vi "Decrypt_Selected_File_of_Hierarchy_Data.vi"(8 "error in (no error)":errorcluster, 9 "FileName":string, 10 "SubFolderName":string, 11 "object in":refnum<class "Crypter.lvclass">) -> (0 "error out":errorcluster, 1 "Folder_Mgmt out":refnum<class "Folder_Mgmt.lvclass">, 2 "Dencrypted text":string, 3 "object out":refnum<class "Crypter.lvclass">)   [LabVIEW 2016, in "Crypter.lvclass"]
uses:
  Crypter.lvclass
  C:/Users/Marco Preziani/Documents/DOME-LV16/WebBrowser_Mgmt/WebBrowser_Mgmt.lvclass
  Folder_Mgmt/Folder_Mgmt.lvclass
  WebBrowser_Mgmt/WebBrowser_Mgmt.lvclass/WebBrowser_Mgmt.ctl
  Folder_Mgmt/Folder_Mgmt.lvclass/Folder_Mgmt.ctl
  WebBrowser_Mgmt/WebBrowser_Mgmt.lvclass
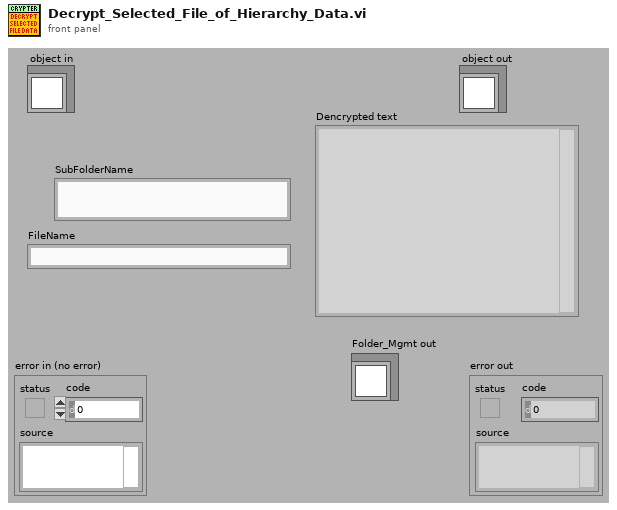
[diagram p1: front panel]
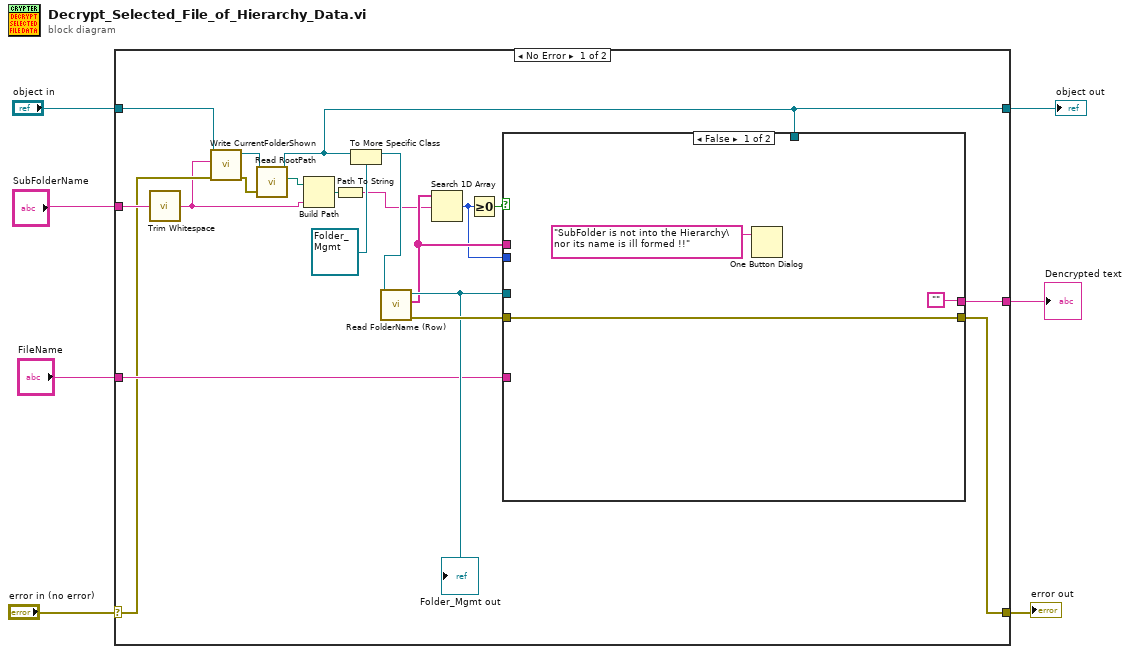
[diagram p0: block diagram]
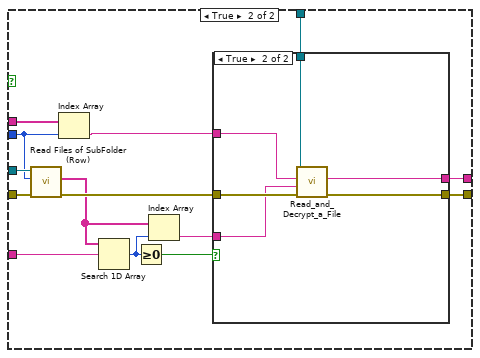
[diagram p2: hidden frame]
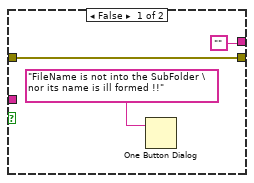
[diagram p3: hidden frame]
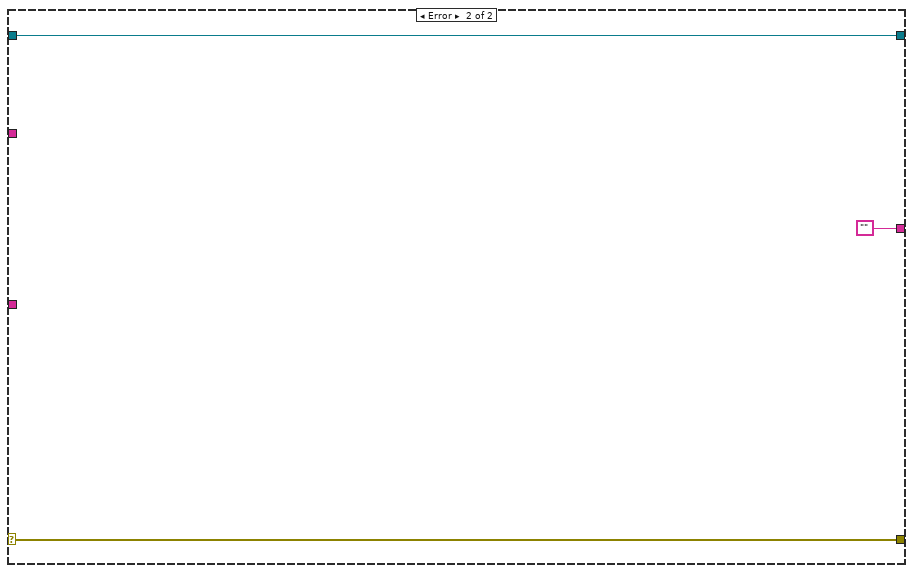
[diagram p4: hidden frame]
diagram:
  n1 = case shown="No Error" "error in (no error)" {
    selector: "error in (no error)" -> [w18 w56]
    tunnel: [w27 w56] -> w6
    tunnel: [w10 w55] -> w4
    tunnel: "object in" -> [w17 w55]
    tunnel: "SubFolderName" -> [w25 _]
    tunnel: "FileName" -> [w20 _]
    tunnel: [w19 ""] -> w1
    frame No Error {
      n2 = call <vilib>:"Trim Whitespace.vi"("string"=w25) -> ("trimmed string"=w12:string)  [unwired: 1 in]
      n3 = call "Write CurrentFolderShown.vi"("error in (no error)"=w18, "CurrentFolderShown"=w12, "WebBrowser_Mgmt in"=w17) -> ("error out"=w8:errorcluster, "WebBrowser_Mgmt out"=w11:refnum<class "Crypter.lvclass">)  [unwired: 7 in]
      n4 = call "Read RootPath.vi"("error in (no error)"=w8, "WebBrowser_Mgmt in"=w11) -> ("RootPath"=w14:path, "WebBrowser_Mgmt out"=w10:refnum<class "Crypter.lvclass">)  [unwired: 7 in, 1 out]
      n5 = Build Path(base path=w14, name or relative path=w12) -> (appended path=w13:path)
      n6 = Path To String(path=w13) -> (string=w9:string)
      n7 = To More Specific Class(target class=refnum<class "Folder_Mgmt.lvclass"> refnum ("Folder_Mgmt.lvclass"), reference=w10) -> (specific class reference=w15:refnum<class "Folder_Mgmt.lvclass">)  [unwired: 1 in, 1 out]
      n8 = call "Read FolderName (Row).vi"("Folder_Mgmt in"=w15) -> ("error out"=w26:errorcluster, "FolderName (Row)"=w23:string[], "Folder_Mgmt out"=w24:refnum<class "Folder_Mgmt.lvclass">)  [unwired: 8 in]
      "Folder_Mgmt out" <- w24
      n9 = Search 1D Array(1D array=w23, element=w9) -> (index of element=w22:i32)  [unwired: 1 in]
      n10 = Greater Or Equal To 0?(x=w22) -> (x >= 0?=w21:bool)
      n11 = case shown="False" w21 {
        tunnel: [w30 w35] -> w27
        tunnel: w26 -> [w30 w44]
        tunnel: w24 -> [_ w43]
        tunnel: w23 -> [_ w41]
        tunnel: w22 -> [_ w34]
        tunnel: w20 -> [_ w39]
        tunnel: ["" w32] -> w19
        tunnel: w10 -> [_ w31]
        frame False {
          n12 = One Button Dialog(message="SubFolder is not into the Hierarchy\nor its name is ill formed !!") -> ()  [unwired: 1 in, 1 out]
        }
        frame True {
          n13 = call "Read Files of SubFolder (Row).vi"("error in (no error)"=w44, "RowIndex"=w34, "Folder_Mgmt in"=w43) -> ("error out"=w42:errorcluster, "FolderFiles (Row)"=w37:string[])  [unwired: 6 in, 1 out]
          n14 = Index Array(array=w41, index=w34) -> (element=w40:string)
          n15 = Search 1D Array(1D array=w37, element=w39) -> (index of element=w38:i32)  [unwired: 1 in]
          n16 = Greater Or Equal To 0?(x=w38) -> (x >= 0?=w33:bool)
          n17 = Index Array(array=w37, index=w38) -> (element=w36:string)
          n18 = case shown="True" w33 {
            tunnel: w42 -> [w46 w53]
            tunnel: w40 -> [_ w52]
            tunnel: w36 -> [_ w51]
            tunnel: [w46 w50] -> w35
            tunnel: ["" w49] -> w32
            tunnel: w31 -> [_ w48]
            frame False {
              n19 = One Button Dialog(message="FileName is not into the SubFolder \nor its name is ill formed !!") -> ()  [unwired: 1 in, 1 out]
            }
            frame True {
              n20 = call-dynamic "Read_and_Decrypt_a_File.vi"("error in (no error)"=w53, "name of File"=w51, "name of Folder"=w52, "object in"=w48) -> ("error out"=w50:errorcluster, "Dencrypted text"=w49:string)  [unwired: 5 in, 1 out]
            }
          }
        }
      }
    }
    frame Error {
    }
  }
  "error out" <- w6
  "object out" <- w4
  "Dencrypted text" <- w1
